vi "Lookup Q by Channel.vi"(8 "error in (no error)":errorcluster, 9 "Timeout ms (5000)":i32=5000, 10 "Channel Name":string, 11 "VolatusAPI in":refnum<class "VolatusAPI.lvclass">) -> (0 "error out":errorcluster, 2 "MessageQ":refnum<class "MessageQ.lvclass">, 3 "VolatusAPI out":refnum<class "VolatusAPI.lvclass">, 5 "Owning Node":string)   [LabVIEW 2020, in "Volatus.lvlib" / "VolatusAPI.lvclass"]
uses:
  VolatusAPI.lvclass
  MessageQ/MessageQ.lvclass
  VolatusAPI.lvclass/VolatusAPI.ctl
  Module Identity/Module Identity.lvclass/Module Identity.ctl
  Module Identity/Module Identity.lvclass
  C:/dev/lv20CE/relink/lv-volatus/Volatus/Identity/Identity.lvclass
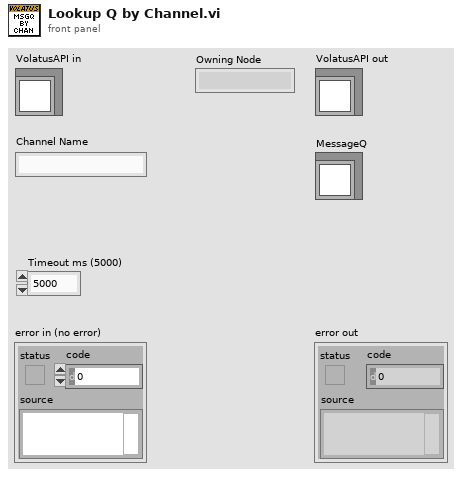
[diagram p1: front panel]
types:
  T1 = typedef "VectoConfig.lvlib/Channel Info.ctl" = cluster{"Name":string, "Group":string, "Owning Node":string, "Owning Task":string, "Resource":string}
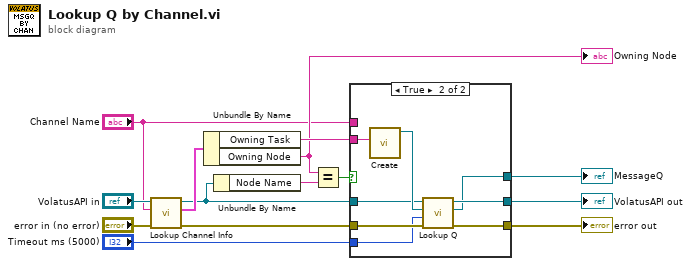
[diagram p0: block diagram]
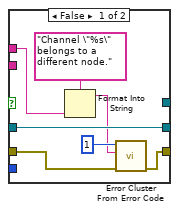
[diagram p2: hidden frame]
diagram:
  n1 = call "Lookup Channel Info.vi"("error in (no error)"="error in (no error)", "Channel Name"="Channel Name", "VolatusAPI in"="VolatusAPI in") -> ("error out"=w14:errorcluster, "Channel Info"=w11:T1, "VolatusAPI out"=w5:refnum<class "VolatusAPI.lvclass">)  [unwired: 4 in, 2 out]
  n2 = Unbundle By Name(w11) -> ("Owning Task"=w10:string, "Owning Node"=w3:string)
  "Owning Node" <- w3
  n3 = Unbundle By Name(w5) -> ("Node Name"=w4:string)
  n4 = Equal?(x=w3, y=w4) -> (x = y?=w2:bool)
  n5 = case shown="True" w2 {
    tunnel: w14 -> [w20 w29]
    tunnel: w10 -> [_ w28]
    tunnel: "Timeout ms (5000)" -> [_ w26]
    tunnel: [w21 w25] -> w8
    tunnel: [w19 w24] -> w7
    tunnel: [_ w23] -> w6
    tunnel: w5 -> [w21 w22]
    tunnel: "Channel Name" -> [w18 _]
    frame False {
      n6 = Format Into String(format string="Channel \"%s\" belongs to a different node.", w18) -> (resulting string=w15:string)  [unwired: 2 in, 1 out]
      n7 = call <vilib>:"Error Cluster From Error Code.vi"("error in (no error)"=w20, "error message (\"\")"=w15, "error code (0)"=1) -> ("error out"=w19:errorcluster)  [unwired: 6 in]
    }
    frame True {
      n8 = call "Create.vi"("ID"=w28) -> ("Module Identity out"=w27:refnum<class "Module Identity.lvclass">)  [unwired: 10 in]
      n9 = call "Lookup Q.vi"("error in (no error)"=w29, "Timeout ms (0)"=w26, "Identity"=w27, "VolatusAPI in"=w22) -> ("error out"=w24:errorcluster, "MessageQ"=w23:refnum<class "MessageQ.lvclass">, "VolatusAPI out"=w25:refnum<class "VolatusAPI.lvclass">)  [unwired: 5 in]
    }
  }
  "error out" <- w7
  "VolatusAPI out" <- w8
  "MessageQ" <- w6
